vi "msg_builder.vi"(9 "constant":string, 10 "comment":string, 11 "type":string) -> (3 "msg":string)   [LabVIEW 2014]
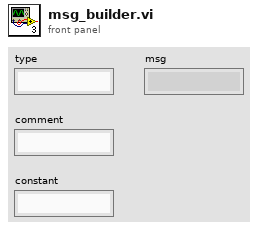
[diagram p1: front panel]
types:
  T1 = cluster{"type":string, "comment":string, "constant":string}
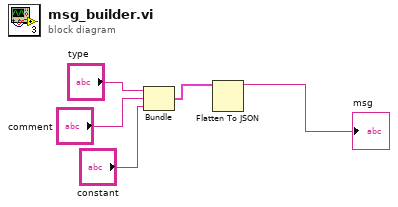
[diagram p0: block diagram]
diagram:
  n1 = Bundle("type"="type", "comment"="comment", "constant"="constant") -> (w4:T1)  [unwired: 1 in]
  n2 = Flatten To JSON(anything=w4) -> (JSON string=→"msg":string)  [unwired: 2 in, 1 out]
